vi "UI.vi"() -> ()   [LabVIEW 2015, in "Editor.lvclass"]
uses:
  Editor.lvclass
  UI_MSG.ctl
  <vilib>/Utility/inputDevices.llb/mouseAcquire.vi
  <vilib>/Utility/inputDevices.llb/closeMouse.vi
  Project.lvclass
  SerializableObject/SerializableObject.lvclass
panel:
  in  "Save As Button":bool
  in  "Save Button":bool
  in  "New Button":bool
  in  "Open Button":bool
  in  "Explorer Tree":string(tree)
  in  "Explorer Drag Receiver":path
  in  "Project Tree":string(tree)
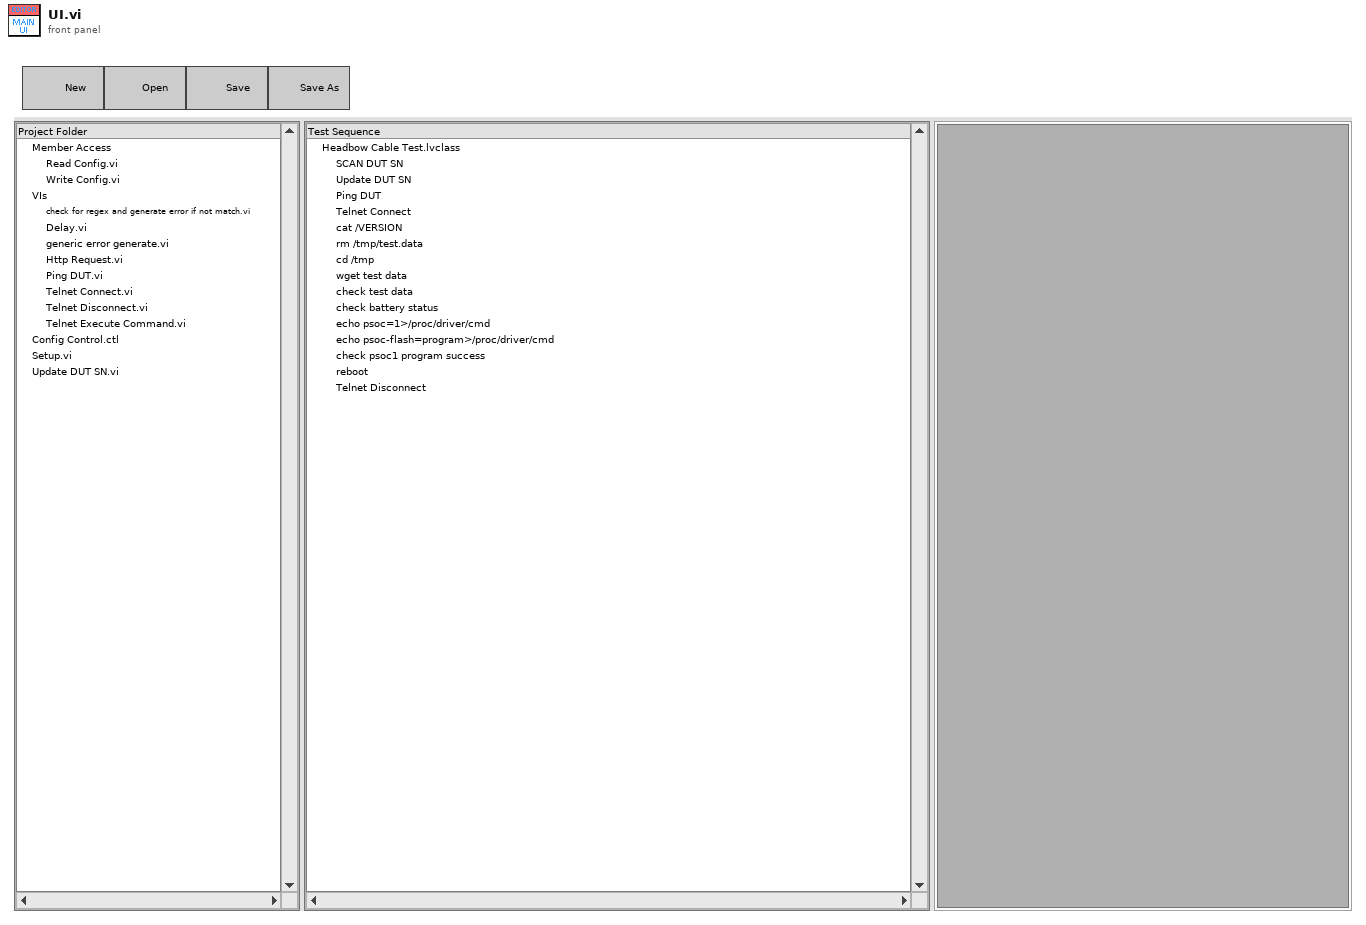
[diagram p1: front panel]
types:
  T1 = typedef "Editor.lvclass/UI_MSG.ctl" = enum16{"EXIT", "INIT_UI", "NEW_PROJECT", "OPEN_PROJECT", "STEP_DISPLAY_UPDATE", "STEP_OPERATION", "UPDATE_UI", "ACTIVE_OBJECT", "DEACTIVE_OBJECT", "SAVE_PROJECT", "ADD_CONFIG"}
  T2 = enum32{"Invalid", "Standard", "Closed", "Hidden", "Minimized", "Maximized"}
  T3 = cluster{"Mode":string, "Source":string, "Target":string}
  T4 = cluster{"Horizontal":i32, "Vertical":i32, "Scrolling":i32}
  T5 = typedef "LVRectTypeDef.ctl" = cluster{"Left":i16, "Top":i16, "Right":i16, "Bottom":i16}
  T6 = cluster{"button 1":bool, "button 2":bool, "button 3":bool, "button 4":bool}
  T7 = typedef "LVPoint32TypeDef.ctl" = cluster{"Horizontal":i32, "Vertical":i32}
  T8 = cluster{"data name":string, "drag data":variant}[]
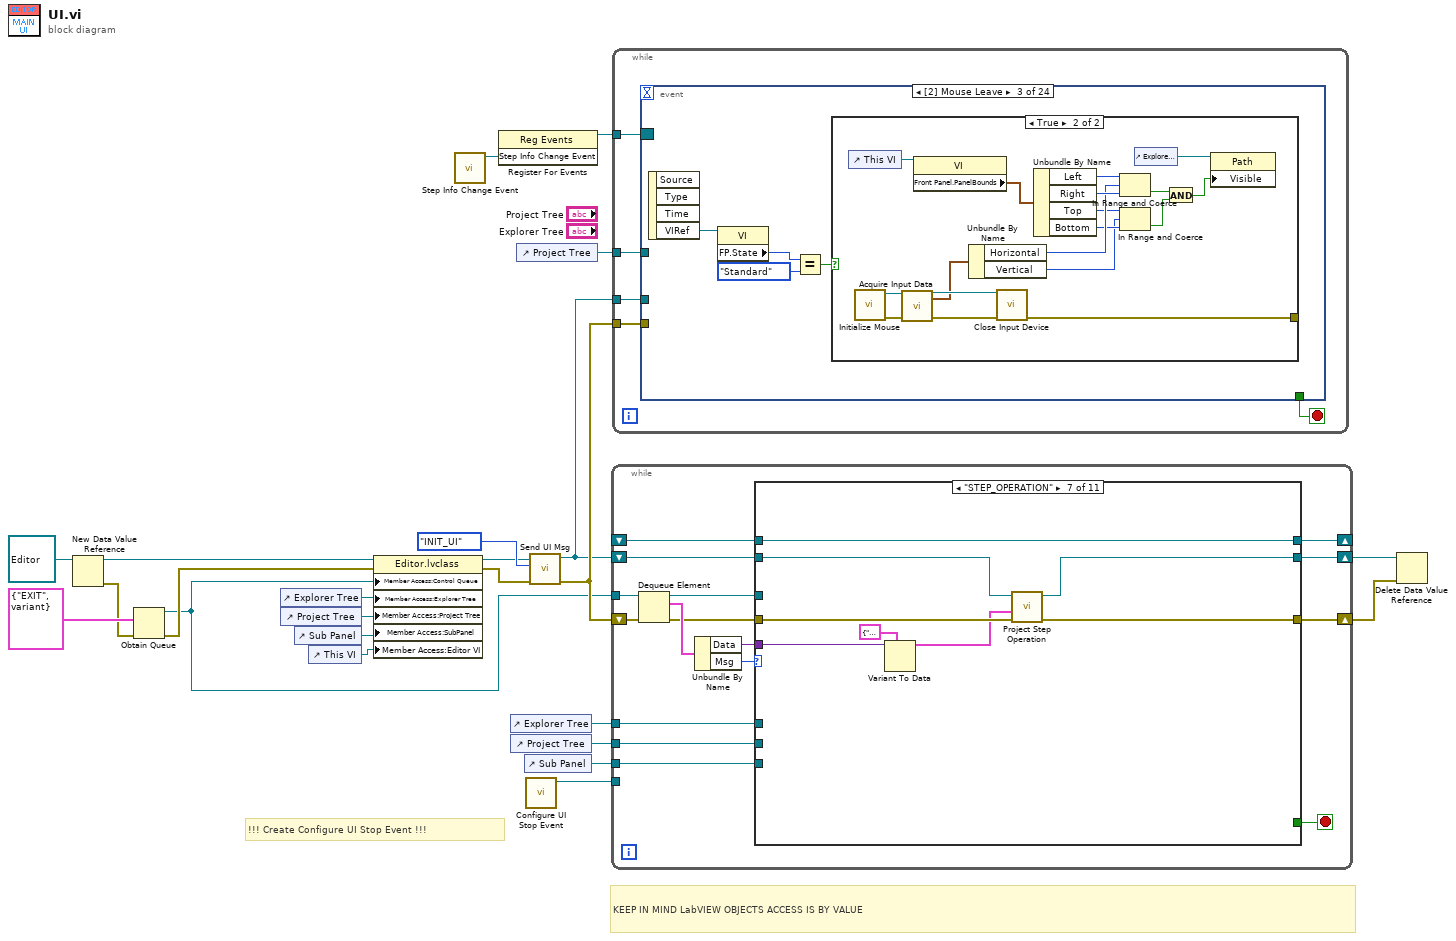
[diagram p0: block diagram]
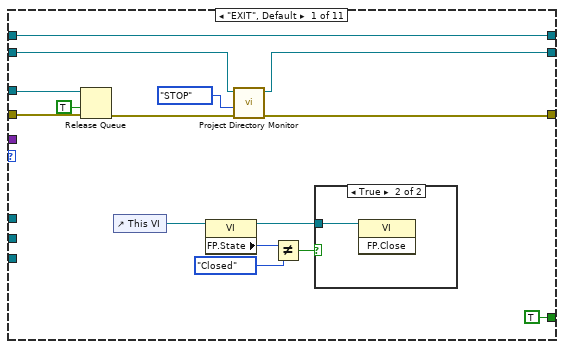
[diagram p2: hidden frame]
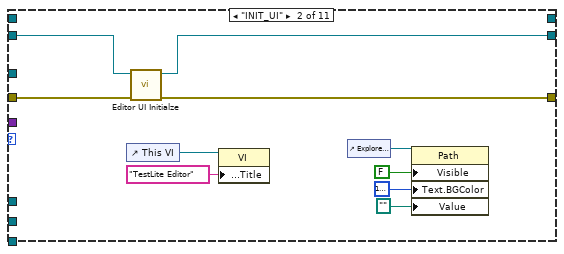
[diagram p4: hidden frame]
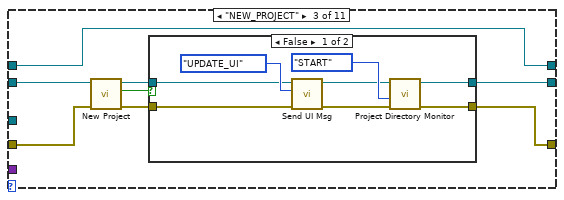
[diagram p5: hidden frame]
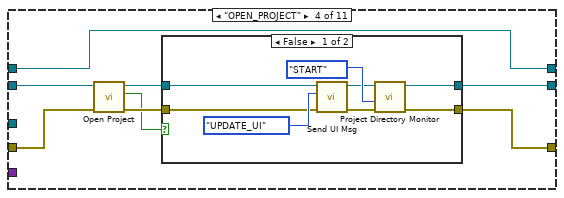
[diagram p7: hidden frame]
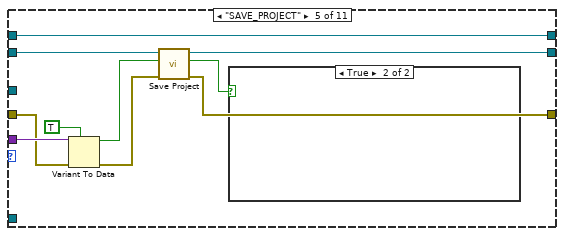
[diagram p9: hidden frame]
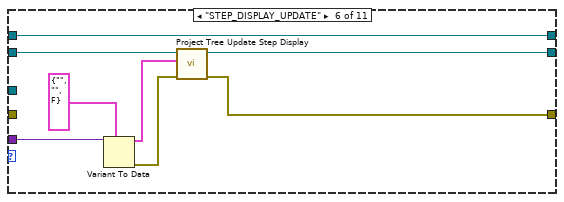
[diagram p11: hidden frame]
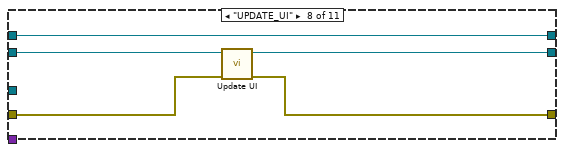
[diagram p12: hidden frame]
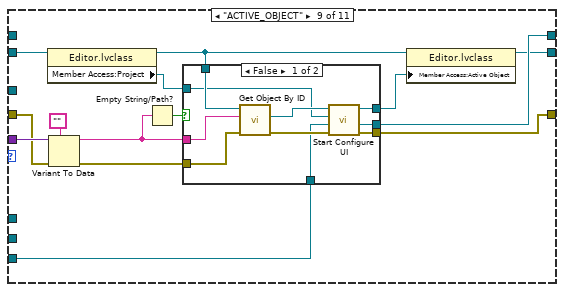
[diagram p13: hidden frame]
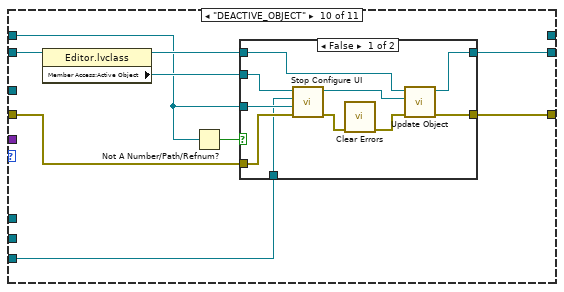
[diagram p15: hidden frame]
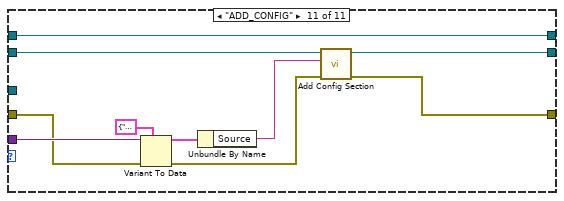
[diagram p17: hidden frame]
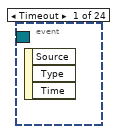
[diagram p18: hidden frame]
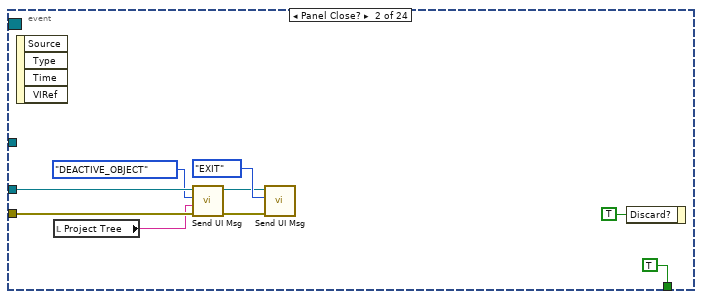
[diagram p19: hidden frame]
diagram:
  # "!!! Create Configure UI Stop Event !!!"
  # "KEEP IN MIND LabVIEW OBJECTS ACCESS IS BY VALUE"
  n1 = New Data Value Reference(data value=refnum<class "Editor.lvclass"> refnum ("Editor.lvclass")) -> (data value reference=w17:refnum<data-value>, error out=w16:errorcluster)  [unwired: 1 in]
  n2 = Obtain Queue(element data type=cluster{"Msg":T1, "Data":variant} {"Msg"=enum."EXIT", "Data"=variant}, error in (no error)=w16) -> (queue out=w9:refnum<queue>, error out=w12:errorcluster)  [unwired: 3 in, 1 out]
  n3 = control-ref of="Explorer Tree"() -> (w15:refnum<vi>)
  n4 = control-ref of="Project Tree"() -> (w14:refnum<vi>)
  n5 = control-ref of="Sub Panel"() -> (w13:refnum<vi>)
  n6 = control-ref of="This VI"() -> (w5:refnum<vi>)
  n7 = property class="Editor.lvclass"(reference=w17, error in=w12, "Member Access:Control Queue"=w9, "Member Access:Explorer Tree"=w15, "Member Access:Project Tree"=w14, "Member Access:SubPanel"=w13, "Member Access:Editor VI"=w5) -> (reference out=w11:refnum<data-value>, error out=w10:errorcluster)
  n8 = call "Step Info Change Event.vi"() -> ("Step Info Change Event"=w4:refnum<user-event>)  [unwired: 11 in]
  n9 = register-events(w4) -> (reference out=w3:refnum<event-registration>)  [unwired: 2 in, 1 out]
  n10 = control-ref of="Explorer Tree"() -> (w19:refnum<vi>)
  n11 = control-ref of="Project Tree"() -> (w20:refnum<vi>)
  n12 = control-ref of="Project Tree"() -> (w1:refnum<vi>)
  n13 = control-ref of="Sub Panel"() -> (w21:refnum<vi>)
  n14 = call "Configure UI Stop Event.vi"() -> ("UI Stop event"=w2:refnum<user-event>)  [unwired: 11 in]
  n15 = call "Send UI Msg.vi"("error in (no error)"=w10, "Msg"=UI_MSG."INIT_UI", "Editor.lvclass in"=w11) -> ("error out"=w23:errorcluster, "Editor.lvclass out"=w8:refnum<data-value>)  [unwired: 7 in]
  n16 = while {
    shift-right: [w34] -> w7
    shift-left: w8 -> [w33]
    tunnel: w9 -> [w39]
    shift-right: [w30] -> w6
    shift-left: w23 -> [w40]
    tunnel: w20 -> [w29]
    tunnel: w21 -> [w28]
    tunnel: w19 -> [w27]
    tunnel: w2 -> [_]
    shift-right: [w26] -> _
    shift-left: _ -> [w25]
    stop <- w35 stop-if-true
    n17 = Dequeue Element(queue=w39, error in (no error)=w40) -> (queue out=w32:refnum<queue>, element=w38:cluster{"Msg":T1, "Data":variant}, error out=w31:errorcluster)  [unwired: 1 in, 1 out]
    n18 = Unbundle By Name(w38) -> ("Data"=w36:variant, "Msg"=w37:T1)
    n19 = case shown="\"STEP_OPERATION\"" w37 {
      tunnel: w36 -> [_ _ _ _ w109 w120 w128 _ w145 _ w185]
      tunnel: [TRUE _ _ _ _ _ _ _ _ _ _] -> w35
      tunnel: [w47 w63 w70 w88 w110 w114 w122 w130 w138 w166 w187] -> w34
      tunnel: w33 -> [w48 w64 w71 w90 w111 w116 w123 w131 w136 w165 w189]
      tunnel: w32 -> [w53 _ _ _ _ _ _ _ _ _ _]
      tunnel: w31 -> [w54 w65 w74 w87 w108 _ w127 w132 w143 w161 w183]
      tunnel: [w50 w66 w72 w92 w112 w115 w126 w133 w147 w167 w186] -> w30
      tunnel: w29 -> [_ _ _ _ _ _ _ _ _ _ _]
      tunnel: w28 -> [_ _ _ _ _ _ _ _ w146 w162 _]
      tunnel: w27 -> [_ _ _ _ _ _ _ _ _ _ _]
      tunnel: [w46 _ w67 w85 w104 w113 w121 w129 w139 _ w188] -> w26
      tunnel: w25 -> [w46 _ w67 w85 w104 w113 w121 w129 _ w160 w188]
      frame "EXIT", Default {
        n20 = Release Queue(queue=w53, force destroy? (F)=TRUE, error in (no error)=w54) -> (error out=w51:errorcluster)  [unwired: 2 out]
        n21 = control-ref of="This VI"() -> (w45:refnum<vi>)
        n22 = property class="VI"(reference=w45) -> (reference out=w41:refnum<vi>, "FP.State"=w44:T2)  [unwired: 1 in, 1 out]
        n23 = call "Project Directory Monitor.vi"("error in (no error)"=w51, "Control"=enum16{"START", "STOP"}."STOP", "Editor.lvclass in"=w48) -> ("error out"=w50:errorcluster, "Editor.lvclass out"=w47:refnum<data-value>)  [unwired: 7 in]
        n24 = Not Equal?(x=w44, y=T2."Closed") -> (x != y?=w42:bool)
        n25 = case shown="True" w42 {
          tunnel: w41 -> [_ w56]
          frame False {
          }
          frame True {
            n26 = invoke class="VI" method="FP.Close"(reference=w56) -> ()  [unwired: 2 in, 3 out]
          }
        }
      }
      frame "INIT_UI" {
        n27 = control-ref of="This VI"() -> (w58:refnum<vi>)
        n28 = call "Editor UI Initialze.vi"("error in (no error)"=w65, "Editor.lvclass in"=w64) -> ("error out"=w66:errorcluster, "Editor.lvclass out"=w63:refnum<data-value>)  [unwired: 8 in]
        n29 = property class="VI"(reference=w58, "Front Panel.Title"="TestLite Editor" ("Front Panel Window:Title")) -> ()  [unwired: 1 in, 2 out]
        n30 = control-ref of="Explorer Drag Receiver"() -> (w62:refnum<vi>)
        n31 = property class="Path"(reference=w62, "Visible"=FALSE, "Text.BGColor"=u32 16777216, "Value"=path "") -> ()  [unwired: 1 in, 2 out]
      }
      frame "NEW_PROJECT" {
        n32 = call "New Project.vi"("error in (no error)"=w74, "Editor.lvclass in"=w71) -> ("error out"=w73:errorcluster, "Cancelled"=w68:bool, "Editor.lvclass out"=w69:refnum<data-value>)  [unwired: 7 in]
        n33 = case shown="False" w68 {
          tunnel: w73 -> [w82 w83]
          tunnel: [w79 w83] -> w72
          tunnel: [w76 w84] -> w70
          tunnel: w69 -> [w75 w84]
          frame False {
            n34 = call "Send UI Msg.vi"("error in (no error)"=w82, "Msg"=UI_MSG."UPDATE_UI", "Editor.lvclass in"=w75) -> ("error out"=w80:errorcluster, "Editor.lvclass out"=w77:refnum<data-value>)  [unwired: 7 in]
            n35 = call "Project Directory Monitor.vi"("error in (no error)"=w80, "Control"=enum16{"START", "STOP"}."START", "Editor.lvclass in"=w77) -> ("error out"=w79:errorcluster, "Editor.lvclass out"=w76:refnum<data-value>)  [unwired: 7 in]
          }
          frame True {
          }
        }
      }
      frame "OPEN_PROJECT" {
        n36 = call "Open Project.vi"("error in (no error)"=w87, "Editor.lvclass in"=w90) -> ("error out"=w91:errorcluster, "Cancelled"=w86:bool, "Editor.lvclass out"=w89:refnum<data-value>)  [unwired: 7 in]
        n37 = case shown="False" w86 {
          tunnel: [w98 w101] -> w92
          tunnel: w91 -> [w96 w101]
          tunnel: w89 -> [w95 w102]
          tunnel: [w93 w102] -> w88
          frame False {
            n38 = call "Send UI Msg.vi"("error in (no error)"=w96, "Msg"=UI_MSG."UPDATE_UI", "Editor.lvclass in"=w95) -> ("error out"=w99:errorcluster, "Editor.lvclass out"=w94:refnum<data-value>)  [unwired: 7 in]
            n39 = call "Project Directory Monitor.vi"("error in (no error)"=w99, "Control"=enum16{"START", "STOP"}."START", "Editor.lvclass in"=w94) -> ("error out"=w98:errorcluster, "Editor.lvclass out"=w93:refnum<data-value>)  [unwired: 7 in]
          }
          frame True {
          }
        }
      }
      frame "SAVE_PROJECT" {
        n40 = Variant To Data(error in=w108, type=TRUE, Variant=w109) -> (data=w105:bool, error out=w106:errorcluster)
        n41 = call "Save Project.vi"("error in (no error)"=w106, "Save As"=w105, "Editor.lvclass in"=w111) -> ("error out"=w112:errorcluster, "Cancelled"=w103:bool, "Editor.lvclass out"=w110:refnum<data-value>)  [unwired: 6 in]
        n42 = case shown="True" w103 {
          frame False {
          }
          frame True {
          }
        }
      }
      frame "STEP_DISPLAY_UPDATE" {
        n43 = Variant To Data(type=cluster{"Id":string, "Name":string, "Skip":bool} {"Id"="", "Name"="", "Skip"=FALSE} ("Step Info"), Variant=w120) -> (data=w118:cluster{"Id":string, "Name":string, "Skip":bool}, error out=w117:errorcluster)  [unwired: 1 in]
        n44 = call "Project Tree Update Step Display.vi"("error in (no error)"=w117, "Step Info"=w118, "Editor.lvclass in"=w116) -> ("error out"=w115:errorcluster, "Editor.lvclass out"=w114:refnum<data-value>)  [unwired: 7 in]
      }
      frame "STEP_OPERATION" {
        n45 = Variant To Data(type=T3 {"Mode"="", "Source"="", "Target"=""} ("Drop Event Data"), Variant=w128) -> (data=w124:T3)  [unwired: 1 in, 1 out]
        n46 = call "Project Step Operation.vi"("error in (no error)"=w127, "Drop Event Data"=w124, "Editor.lvclass in"=w123) -> ("error out"=w126:errorcluster, "Editor.lvclass out"=w122:refnum<data-value>)  [unwired: 7 in]
      }
      frame "UPDATE_UI" {
        n47 = call "Update UI.vi"("error in (no error)"=w132, "Editor.lvclass in"=w131) -> ("error out"=w133:errorcluster, "Editor.lvclass out"=w130:refnum<data-value>)  [unwired: 8 in]
      }
      frame "ACTIVE_OBJECT" {
        n48 = property class="Editor.lvclass"(reference=w136) -> (reference out=w135:refnum<data-value>, "Member Access:Project"=w134:refnum<class "Project.lvclass">)  [unwired: 1 in, 1 out]
        n49 = Variant To Data(error in=w143, type="", Variant=w145) -> (data=w141:string, error out=w142:errorcluster)
        n50 = Empty String/Path?(string/path=w141) -> (empty?=w140:bool)
        n51 = case shown="False" w140 {
          tunnel: [w152 w158] -> w147
          tunnel: w146 -> [w149 _]
          tunnel: w141 -> [w157 _]
          tunnel: w142 -> [w156 w158]
          tunnel: w135 -> [w155 _]
          tunnel: [w153 _] -> w137
          tunnel: [w150 _] -> w139
          tunnel: w134 -> [w148 _]
          frame False {
            n52 = call "Get Object By ID.vi"("error in (no error)"=w156, "ID"=w157, "Editor.lvclass in"=w155) -> ("error out"=w151:errorcluster, "SerializableObject out"=w154:refnum<class "SerializableObject.lvclass">)  [unwired: 6 in, 1 out]
            n53 = call "Start Configure UI.vi"("error in (no error)"=w151, "Container"=w149, "Project In"=w148, "SerializableObject in"=w154) -> ("error out"=w152:errorcluster, "Configure VI Refnum"=w150:refnum<vi>, "SerializableObject out"=w153:refnum<class "SerializableObject.lvclass">)  [unwired: 5 in]
          }
          frame True {
          }
        }
        n54 = property class="Editor.lvclass"(reference=w135, "Member Access:Active Object"=w137) -> (reference out=w138:refnum<data-value>)  [unwired: 1 in, 1 out]
      }
      frame "DEACTIVE_OBJECT" {
        n55 = property class="Editor.lvclass"(reference=w165) -> (reference out=w164:refnum<data-value>, "Member Access:Active Object"=w163:refnum<class "SerializableObject.lvclass">)  [unwired: 1 in, 1 out]
        n56 = Not A Number/Path/Refnum?(number/path/refnum=w160) -> (NaN/Path/Refnum?=w159:bool)
        n57 = case shown="False" w159 {
          tunnel: w161 -> [w171 w178]
          tunnel: [w177 w178] -> w167
          tunnel: w164 -> [w175 w179]
          tunnel: [w176 w179] -> w166
          tunnel: w163 -> [w173 _]
          tunnel: w160 -> [w169 _]
          tunnel: w162 -> [w168 _]
          frame False {
            n58 = call "Stop Configure UI.vi"("error in (no error)"=w171, "Configure VI Refnum"=w169, "Container"=w168, "SerializableObject in"=w173) -> ("error out"=w170:errorcluster, "SerializableObject out"=w172:refnum<class "SerializableObject.lvclass">)  [unwired: 6 in]
            n59 = call <vilib>:"Clear Errors.vi"("error in (no error)"=w170) -> ("error out"=w174:errorcluster)  [unwired: 5 in, 1 out]
            n60 = call "Update Object.vi"("error in (no error)"=w174, "SerializableObject in"=w172, "Editor.lvclass in"=w175) -> ("error out"=w177:errorcluster, "Editor.lvclass out"=w176:refnum<data-value>)  [unwired: 7 in]
          }
          frame True {
          }
        }
      }
      frame "ADD_CONFIG" {
        n61 = Variant To Data(error in=w183, type=T3 {"Mode"="", "Source"="", "Target"=""} ("Drop Event Data"), Variant=w185) -> (data=w181:T3, error out=w182:errorcluster)
        n62 = Unbundle By Name(w181) -> ("Source"=w180:string)
        n63 = call "Add Config Section.vi"("error in (no error)"=w182, "FileName"=w180, "Editor.lvclass in"=w189) -> ("error out"=w186:errorcluster, "Editor.lvclass out"=w187:refnum<data-value>)  [unwired: 7 in]
      }
    }
  }
  n64 = while {
    tunnel: w8 -> [w193]
    tunnel: w23 -> [w192]
    tunnel: w3 -> [w191]
    tunnel: w1 -> [w190]
    stop <- w194 stop-if-true
    n65 = event shown="[2] Mouse Leave" {
      selector: w191 -> [_ _ _ _ _ _ _ _ _ _ _ _ _ _ _ _ _ _ _ _ _ _ _ _]
      dyn-events: _ -> [_ _ _ _ _ _ _ _ _ _ _ _ _ _ _ _ _ _ _ _ _ _ _ _]
      timeout: _ -> [_ _ _ _ _ _ _ _ _ _ _ _ _ _ _ _ _ _ _ _ _ _ _ _]
      tunnel: [_ TRUE _ _ _ _ _ _ _ _ _ _ _ _ _ _ _ _ _ _ _ _ _ _] -> w194
      tunnel: w193 -> [_ w200 _ _ w240 _ _ _ _ w288 _ _ w311 _ w344 _ _ w372 w386 w391 w398 w406 w408 w418]
      tunnel: w192 -> [_ w199 _ _ w237 _ _ _ _ w291 _ _ w310 _ w343 _ _ w371 w385 w390 w397 w405 w407 w417]
      tunnel: w190 -> [_ _ _ _ w236 _ _ _ _ _ _ _ _ _ _ _ _ _ _ _ _ _ _ _]
      event Timeout {
        n66 = event-data() -> ()  [unwired: 1 in, 3 out]
      }
      event Panel Close? {
        n67 = event-data() -> ()  [unwired: 1 in, 4 out]
        n68 = local read "Project Tree"() -> (w195:string)
        n69 = call "Send UI Msg.vi"("error in (no error)"=w199, "Data"=w195, "Msg"=UI_MSG."DEACTIVE_OBJECT", "Editor.lvclass in"=w200) -> ("error out"=w197:errorcluster, "Editor.lvclass out"=w198:refnum<data-value>)  [unwired: 6 in]
        n70 = call "Send UI Msg.vi"("error in (no error)"=w197, "Msg"=UI_MSG."EXIT", "Editor.lvclass in"=w198) -> ()  [unwired: 7 in, 2 out]
        n71 = event-data("Discard?"=TRUE) -> ()  [unwired: 1 in, 1 out]
      }
      event Mouse Leave {
        n72 = event-data() -> ("VIRef"=w207:refnum<vi>)  [unwired: 1 in, 3 out]
        n73 = property class="VI"(reference=w207) -> ("FP.State"=w206:T2)  [unwired: 1 in, 2 out]
        n74 = Equal?(x=w206, y=T2."Standard") -> (x = y?=w204:bool)
        n75 = case shown="True" w204 {
          tunnel: [_ w208] -> _
          frame False {
          }
          frame True {
            n76 = control-ref of="This VI"() -> (w219:refnum<vi>)
            n77 = call <vilib>:"Initialize Mouse.vi"() -> ("error out"=w223:errorcluster, "device ID"=w222:refnum<k1>)  [unwired: 1 in, 9 out]
            n78 = call-poly <vilib>:"Acquire Input Data.vi"("device ID"=w222, "error in (no error)"=w223) -> ("device ID"=w221:refnum<k1>, "axis info"=w218:T4, "error out"=w224:errorcluster)  [unwired: 1 in, 14 out]
            n79 = property class="VI"(reference=w219) -> ("Front Panel.PanelBounds"=w220:T5)  [unwired: 1 in, 2 out]
            n80 = Unbundle By Name(w218) -> ("Horizontal"=w215:i32, "Vertical"=w212:i32)
            n81 = call-poly <vilib>:"Close Input Device.vi"("error in (no error)"=w224, "device ID"=w221) -> ("error out"=w208:errorcluster)  [unwired: 8 out]
            n82 = Unbundle By Name(w220) -> ("Left"=w217:i16, "Right"=w216:i16, "Top"=w214:i16, "Bottom"=w213:i16)
            n83 = In Range and Coerce(upper limit=w217, x=w215, lower limit=w216) -> (In Range?=w211:bool)  [unwired: 1 out]
            n84 = In Range and Coerce(upper limit=w214, x=w212, lower limit=w213) -> (In Range?=w210:bool)  [unwired: 1 out]
            n85 = control-ref of="Explorer Drag Receiver"() -> (w225:refnum<vi>)
            n86 = And(x=w211, y=w210) -> (x .and. y?=w209:bool)
            n87 = property class="Path"(reference=w225, "Visible"=w209) -> ()  [unwired: 1 in, 2 out]
          }
        }
      }
      event Mouse Enter {
        n88 = event-data() -> ()  [unwired: 1 in, 4 out]
        n89 = call <vilib>:"Initialize Mouse.vi"() -> ("error out"=w229:errorcluster, "device ID"=w228:refnum<k1>)  [unwired: 1 in, 9 out]
        n90 = call-poly <vilib>:"Acquire Input Data.vi"("device ID"=w228, "error in (no error)"=w229) -> ("device ID"=w231:refnum<k1>, "button info"=w227:T6, "error out"=w230:errorcluster)  [unwired: 1 in, 14 out]
        n91 = Unbundle By Name(w227) -> ("button 1"=w226:bool)
        n92 = call-poly <vilib>:"Close Input Device.vi"("error in (no error)"=w230, "device ID"=w231) -> ()  [unwired: 9 out]
        n93 = case shown="False" w226 {
          frame False {
            n94 = control-ref of="Explorer Drag Receiver"() -> (w233:refnum<vi>)
            n95 = property class="Path"(reference=w233, "Visible"=FALSE, "Value"=path "") -> ()  [unwired: 1 in, 2 out]
          }
          frame True {
          }
        }
      }
      event Key Down? {
        n96 = event-data() -> ("ScanCode"=w235:i16, "PlatMods.Ctrl"=w241:bool)  [unwired: 1 in]
        n97 = property on="Project Tree" class="Tree (strict)"() -> ("Key Focus"=w238:bool)  [unwired: 2 in, 2 out]
        n98 = case shown="True" w238 {
          tunnel: w235 -> [_ w249]
          tunnel: w241 -> [_ w248]
          tunnel: w240 -> [_ w247]
          tunnel: [_ w245] -> w239
          tunnel: w237 -> [_ w244]
          tunnel: w236 -> [_ w242]
          frame False {
          }
          frame True {
            n99 = call "Project Tree Process Keydown Event.vi"("Project Tree"=w242, "Ctrl"=w248, "ScanCode"=w249) -> ("Step Operation Data"=w243:T3, "Operation Accept"=w246:bool, "Event Discard"=w245:bool)  [unwired: 6 in]
            n100 = case shown="True" w246 {
              tunnel: w243 -> [_ w255]
              tunnel: w247 -> [_ w254]
              tunnel: w244 -> [_ w250]
              frame False {
              }
              frame True {
                n101 = call "Send UI Msg.vi"("error in (no error)"=w250, "Msg"=UI_MSG."DEACTIVE_OBJECT", "Editor.lvclass in"=w254) -> ("error out"=w253:errorcluster, "Editor.lvclass out"=w252:refnum<data-value>)  [unwired: 7 in]
                n102 = call "Send UI Msg.vi"("error in (no error)"=w253, "Data"=w255, "Msg"=UI_MSG."STEP_OPERATION", "Editor.lvclass in"=w252) -> ()  [unwired: 6 in, 2 out]
              }
            }
          }
        }
        n103 = event-data("Discard?"=w239) -> ()  [unwired: 1 in, 1 out]
      }
      event "Project Tree": Drag Starting? {
        n104 = event-data() -> ("PlatMods.Ctrl"=w260:bool, "CtlRef"=w268:refnum<vi>, "Coords"=w267:T7)  [unwired: 1 in]
        n105 = invoke class="Tree (strict)" method="Point To Row Column"(reference=w268, "Point"=w267) -> ("Tag"=w266:string)  [unwired: 6 in, 7 out]
        n106 = Select(t=enum32{"copy or move", "copy only", "move only"}."copy only" ("Drag Mode"), s=w260, f=enum32{"copy or move", "copy only", "move only"}."move only" ("Drag Mode")) -> (s? t:f=w257:enum32{"copy or move", "copy only", "move only"})
        n107 = Select(t="COPY", s=w260, f="MOVE") -> (s? t:f=w263:string)
        n108 = call "Build Drag Data.vi"("Source"=w266, "Mode"=w263) -> ("Drag Data"=w262:T8)  [unwired: 2 in]
        n109 = event-data("Drag Mode"=w257, "Data"=w262, "Discard?"=FALSE) -> ()  [unwired: 1 in, 1 out]
      }
      event "Project Tree": Drag Ended {
        n110 = event-data() -> ("CtlRef"=w269:refnum<vi>, "Result"=w270:enum16{"Drop Cancel", "Drop Move", "Drop Copy"})  [unwired: 1 in]
        n111 = case shown="\"Drop Cancel\"" w270 {
          tunnel: w269 -> [_ w273]
          frame Default {
          }
          frame "Drop Cancel" {
            n112 = property class="Tree (strict)"(reference=w273) -> (reference out=w272:refnum<vi>, "All Tags"=w271:string[])  [unwired: 1 in, 1 out]
            n113 = for {
              tunnel: w272 -> [w277]
              tunnel: w271 -> [w276] mode=indexing
              n114 = property class="Tree (strict)"(reference=w277, "Active Item Tag"=w276, "ActiveColNum"=0 ("Active Cell:Active Column Number"), "CellBG"=u32 16777216) -> ()  [unwired: 1 in, 2 out]
            }
          }
        }
      }
      event "Project Tree": Drag Enter {
        n115 = event-data() -> ("Available Data Names"=w281:string[])  [unwired: 1 in]
        n116 = Search 1D Array(1D array=w281, element="DragData" ("data name")) -> (index of element=w279:i32)  [unwired: 1 in]
        n117 = Greater Or Equal To 0?(x=w279) -> (x >= 0?=w278:bool)
        n118 = event-data("Accepted?"=w278) -> ()  [unwired: 1 in, 1 out]
      }
      event "Project Tree": event type 3.0.xa000003a {
        n119 = event-data() -> ("CtlRef"=w285:refnum<vi>, "Coords"=w284:T7, "Available Data Names"=w283:string[])  [unwired: 1 in]
        n120 = call "Project Tree Drag Over.vi"("Available Data Names"=w283, "Coords"=w284, "TreeControl in"=w285) -> ("Accepted"=w282:bool)  [unwired: 6 in, 2 out]
        n121 = event-data("Accepted?"=w282) -> ()  [unwired: 1 in, 1 out]
      }
      event "Project Tree": Drop {
        # "Deactive current object, otherwise you will lost all changes\nEspecially if current active item is project"
        n122 = event-data() -> ("CtlRef"=w292:refnum<vi>, "Coords"=w293:T7, "Available Data Names"=w294:string[])  [unwired: 1 in]
        n123 = call "Project Tree Drop.vi"("error in (no error)"=w291, "Available Data Names"=w294, "Coords"=w293, "TreeControl in"=w292) -> ("error out"=w289:errorcluster, "Step Operation Data"=w290:T3, "Valid"=w286:bool)  [unwired: 5 in]
        n124 = case shown="True" w286 {
          tunnel: w290 -> [_ w300]
          tunnel: w289 -> [_ w298]
          tunnel: w288 -> [_ w299]
          tunnel: [_ FALSE] -> w287
          frame False {
          }
          frame True {
            n125 = call "Send UI Msg.vi"("error in (no error)"=w298, "Msg"=UI_MSG."DEACTIVE_OBJECT", "Editor.lvclass in"=w299) -> ("error out"=w297:errorcluster, "Editor.lvclass out"=w296:refnum<data-value>)  [unwired: 7 in]
            n126 = call "Send UI Msg.vi"("error in (no error)"=w297, "Data"=w300, "Msg"=UI_MSG."STEP_OPERATION", "Editor.lvclass in"=w296) -> ()  [unwired: 6 in, 2 out]
          }
        }
        n127 = event-data("Accepted?"=w287) -> ()  [unwired: 1 in, 1 out]
      }
      event "Project Tree": Shortcut Menu Activation? {
        n128 = event-data() -> ("CtlRef"=w306:refnum<vi>, "MenuRef"=w305:refnum<k9>, "Coords"=w304:T7)  [unwired: 1 in]
        n129 = call "Build Project Tree Menu.vi"("Coords"=w304, "Project Tree Menu"=w305, "Project Tree"=w306) -> ("Discard"=w303:bool)  [unwired: 8 in]
        n130 = event-data("Discard?"=w303) -> ()  [unwired: 1 in, 1 out]
      }
      event "Project Tree": event #0x44 {
        n131 = event-data() -> ()  [unwired: 1 in, 4 out]
        n132 = control-ref of="Explorer Drag Receiver"() -> (w308:refnum<vi>)
        n133 = property class="Path"(reference=w308, "Visible"=FALSE, "Value"=path "") -> ()  [unwired: 1 in, 2 out]
      }
      event "Project Tree": Shortcut Menu Selection (User) {
        n134 = event-data() -> ("ItemTag"=w312:string)  [unwired: 1 in]
        n135 = case shown="\"ADD_EXE_STEP\", \"ADD_UI_STEP\", \"ADD_VI_STEP\", \"REMOVE\"" w312 {
          selector: w312 -> [_ w313]
          tunnel: w311 -> [_ w316]
          tunnel: w310 -> [_ w315]
          frame Default {
          }
          frame "ADD_EXE_STEP", "ADD_UI_STEP", "ADD_VI_STEP", "REMOVE" {
            n136 = local read "Project Tree"() -> (w314:string)
            n137 = Bundle By Name(cluster=T3 {"Mode"="", "Source"="", "Target"=""} ("Drop Event Data"), "Mode"=w313, "Source"=w314) -> (w320:T3)
            n138 = call "Send UI Msg.vi"("error in (no error)"=w315, "Data"=w314, "Msg"=UI_MSG."DEACTIVE_OBJECT", "Editor.lvclass in"=w316) -> ("error out"=w319:errorcluster, "Editor.lvclass out"=w318:refnum<data-value>)  [unwired: 6 in]
            n139 = call "Send UI Msg.vi"("error in (no error)"=w319, "Data"=w320, "Msg"=UI_MSG."STEP_OPERATION", "Editor.lvclass in"=w318) -> ()  [unwired: 6 in, 2 out]
          }
        }
      }
      event "Explorer Tree": Drag Starting? {
        n140 = event-data() -> ("CtlRef"=w332:refnum<vi>)  [unwired: 1 in]
        n141 = property class="Tree (strict)"(reference=w332) -> ("Value"=w324:string)  [unwired: 1 in, 2 out]
        n142 = String To Path(string=w324) -> (path=w328:path)
        n143 = call <vilib>:"Get File Extension.vi"("file"=w328) -> ("lowercase file extension"=w326:string)  [unwired: 6 in, 4 out]
        n144 = Search 1D Array(1D array=string[] ["vi", "exe"], element=w326) -> (index of element=w325:i32)  [unwired: 1 in]
        n145 = Greater Or Equal To 0?(x=w325) -> (x >= 0?=w323:bool)
        n146 = case shown="False" w323 {
          tunnel: [_ enum32{"copy or move", "copy only", "move only"}."copy only" ("Drag Mode")] -> w331
          tunnel: [TRUE FALSE ("Discard?")] -> w330
          tunnel: [_ w335] -> w329
          tunnel: w324 -> [_ w334]
          frame False {
          }
          frame True {
            n147 = call "Build Drag Data.vi"("Source"=w334, "Mode"="NEW") -> ("Drag Data"=w335:T8)  [unwired: 2 in]
          }
        }
        n148 = event-data("Data"=w329, "Drag Mode"=w331, "Discard?"=w330) -> ()  [unwired: 1 in, 1 out]
      }
      event "Explorer Drag Receiver": Value Change {
        n149 = event-data() -> ("NewVal"=w342:path)  [unwired: 1 in]
        n150 = call <vilib>:"Check if File or Folder Exists.vi"("path"=w342) -> ("error out"=w339:errorcluster, "file or folder exists?"=w340:bool, "dup path"=w341:path)  [unwired: 8 in]
        n151 = case shown="True" w340 {
          tunnel: w344 -> [_ w351]
          tunnel: w343 -> [_ w350]
          tunnel: w341 -> [_ w348]
          tunnel: w339 -> [_ w347]
          frame False {
            n152 = One Button Dialog(message="File must exist!") -> ()  [unwired: 1 in, 1 out]
          }
          frame True {
            n153 = call <vilib>:"Get File Extension.vi"("error in (no error)"=w347, "file"=w348) -> ("lowercase file extension"=w346:string, "dup file"=w349:path)  [unwired: 5 in, 3 out]
            n154 = case shown="\"exe\", \"vi\"" w346 {
              tunnel: w351 -> [_ w358]
              tunnel: w350 -> [_ w357]
              tunnel: w349 -> [_ w353]
              frame Default {
                n155 = One Button Dialog(message="Only VI or EXE file acceptable!") -> ()  [unwired: 1 in, 1 out]
              }
              frame "exe", "vi" {
                n156 = Path To String(path=w353) -> (string=w360:string)
                n157 = Bundle By Name(cluster=T3 {"Mode"="", "Source"="", "Target"=""} ("Drop Event Data"), "Mode"="NEW", "Source"=w360) -> (w359:T3)
                n158 = call "Send UI Msg.vi"("error in (no error)"=w357, "Msg"=UI_MSG."DEACTIVE_OBJECT", "Editor.lvclass in"=w358) -> ("error out"=w356:errorcluster, "Editor.lvclass out"=w355:refnum<data-value>)  [unwired: 7 in]
                n159 = call "Send UI Msg.vi"("error in (no error)"=w356, "Data"=w359, "Msg"=UI_MSG."STEP_OPERATION", "Editor.lvclass in"=w355) -> ()  [unwired: 6 in, 2 out]
              }
            }
          }
        }
      }
      event "Explorer Tree": Shortcut Menu Activation? {
        n160 = event-data() -> ("CtlRef"=w367:refnum<vi>, "MenuRef"=w366:refnum<k9>, "Coords"=w365:T7)  [unwired: 1 in]
        n161 = call "Build Project Directory Menu.vi"("Coords"=w365, "Project Tree Menu"=w366, "Project Tree"=w367) -> ("Discard"=w364:bool)  [unwired: 8 in]
        n162 = event-data("Discard?"=w364) -> ()  [unwired: 1 in, 1 out]
      }
      event "Explorer Tree": event #0x44 {
        n163 = event-data() -> ()  [unwired: 1 in, 4 out]
        n164 = control-ref of="Explorer Drag Receiver"() -> (w369:refnum<vi>)
        n165 = property class="Path"(reference=w369, "Visible"=FALSE, "Value"=path "") -> ()  [unwired: 1 in, 2 out]
      }
      event "Explorer Tree": Shortcut Menu Selection (User) {
        n166 = event-data() -> ("ItemTag"=w373:string)  [unwired: 1 in]
        n167 = case shown="\"ADD_CONFIG\"" w373 {
          selector: w373 -> [_ w379]
          tunnel: w372 -> [_ w376]
          tunnel: w371 -> [_ w375]
          frame Default {
          }
          frame "ADD_CONFIG" {
            n168 = local read "Explorer Tree"() -> (w378:string)
            n169 = Bundle By Name(cluster=T3 {"Mode"="", "Source"="", "Target"=""} ("Drop Event Data"), "Mode"=w379, "Source"=w378) -> (w377:T3)
            n170 = call "Send UI Msg.vi"("error in (no error)"=w375, "Data"=w377, "Msg"=UI_MSG."ADD_CONFIG", "Editor.lvclass in"=w376) -> ()  [unwired: 6 in, 2 out]
          }
        }
      }
      event "Project Tree": Value Change {
        n171 = event-data() -> ("NewVal"=w387:string, "OldVal"=w381:string)  [unwired: 1 in]
        n172 = call "Send UI Msg.vi"("error in (no error)"=w385, "Data"=w381, "Msg"=UI_MSG."DEACTIVE_OBJECT", "Editor.lvclass in"=w386) -> ("error out"=w383:errorcluster, "Editor.lvclass out"=w384:refnum<data-value>)  [unwired: 6 in]
        n173 = call "Send UI Msg.vi"("error in (no error)"=w383, "Data"=w387, "Msg"=UI_MSG."ACTIVE_OBJECT", "Editor.lvclass in"=w384) -> ()  [unwired: 6 in, 2 out]
      }
      event "New Button": Value Change {
        n174 = event-data() -> ()  [unwired: 1 in, 2 out]
        n175 = call "Send UI Msg.vi"("error in (no error)"=w390, "Msg"=UI_MSG."NEW_PROJECT", "Editor.lvclass in"=w391) -> ()  [unwired: 7 in, 2 out]
      }
      event "Open Button": Value Change {
        n176 = event-data() -> ()  [unwired: 1 in, 2 out]
        n177 = local read "Project Tree"() -> (w395:string)
        n178 = call "Send UI Msg.vi"("error in (no error)"=w397, "Data"=w395, "Msg"=UI_MSG."DEACTIVE_OBJECT", "Editor.lvclass in"=w398) -> ("error out"=w394:errorcluster, "Editor.lvclass out"=w393:refnum<data-value>)  [unwired: 6 in]
        n179 = call "Send UI Msg.vi"("error in (no error)"=w394, "Msg"=UI_MSG."OPEN_PROJECT", "Editor.lvclass in"=w393) -> ()  [unwired: 7 in, 2 out]
      }
      event "Save Button": Value Change {
        n180 = event-data() -> ()  [unwired: 1 in, 1 out]
        n181 = local read "Project Tree"() -> (w403:string)
        n182 = call "Send UI Msg.vi"("error in (no error)"=w405, "Data"=w403, "Msg"=UI_MSG."DEACTIVE_OBJECT", "Editor.lvclass in"=w406) -> ("error out"=w402:errorcluster, "Editor.lvclass out"=w401:refnum<data-value>)  [unwired: 6 in]
        n183 = call "Send UI Msg.vi"("error in (no error)"=w402, "Data"=FALSE, "Msg"=UI_MSG."SAVE_PROJECT", "Editor.lvclass in"=w401) -> ()  [unwired: 6 in, 2 out]
      }
      event "Save As Button": Value Change {
        n184 = event-data() -> ()  [unwired: 1 in, 6 out]
        n185 = local read "Project Tree"() -> (w413:string)
        n186 = call "Send UI Msg.vi"("error in (no error)"=w407, "Data"=w413, "Msg"=UI_MSG."DEACTIVE_OBJECT", "Editor.lvclass in"=w408) -> ("error out"=w412:errorcluster, "Editor.lvclass out"=w411:refnum<data-value>)  [unwired: 6 in]
        n187 = call "Send UI Msg.vi"("error in (no error)"=w412, "Data"=TRUE, "Msg"=UI_MSG."SAVE_PROJECT", "Editor.lvclass in"=w411) -> ()  [unwired: 6 in, 2 out]
      }
      event User Event {
        n188 = event-data() -> ("Value"=w420:variant)  [unwired: 1 in]
        n189 = Variant To Data(type=cluster{"Id":string, "Name":string, "Skip":bool} {"Id"="", "Name"="", "Skip"=FALSE} ("Step Info"), Variant=w420) -> (data=w415:cluster{"Id":string, "Name":string, "Skip":bool})  [unwired: 1 in, 1 out]
        n190 = call "Send UI Msg.vi"("error in (no error)"=w417, "Data"=w415, "Msg"=UI_MSG."STEP_DISPLAY_UPDATE", "Editor.lvclass in"=w418) -> ()  [unwired: 6 in, 2 out]
      }
    }
  }
  n191 = Delete Data Value Reference(data value reference=w7, error in=w6) -> ()  [unwired: 2 out]
